vi "Error Handler Loop.vi"(8 "error in (no error)":errorcluster) -> (0 "error out":errorcluster)   [LabVIEW 2018, in "Error Handler.lvlib"]
uses:
  Error Handler.lvlib
  Q Ref FGV Command Enum.ctl
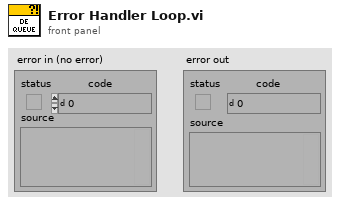
[diagram p1: front panel]
types:
  T1 = typedef "Error Handler.lvlib/Q Ref FGV Command Enum.ctl" = enum16{"Create Q", "Get Q", "Flush Q", "Release Q"}
  T2 = cluster{"Source":string, "Error to Handle":errorcluster}
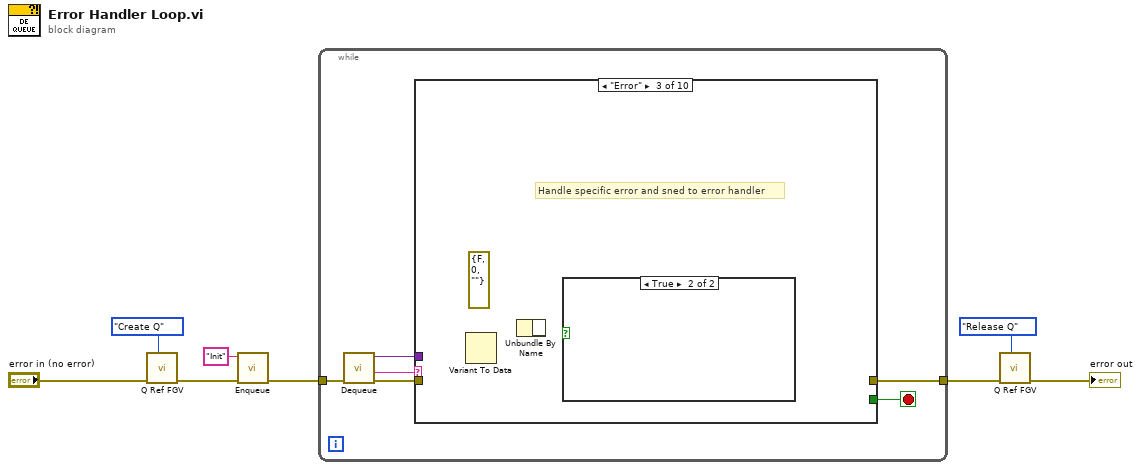
[diagram p0: block diagram]
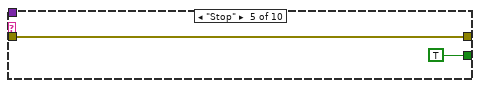
[diagram p6: hidden frame]
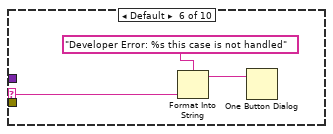
[diagram p7: hidden frame]
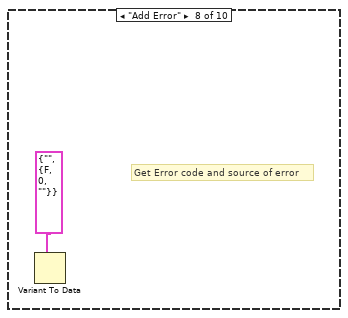
[diagram p9: hidden frame]
diagram:
  n1 = call "Q Ref FGV.vi"("Command"=Q_Ref_FGV_Command_Enum."Create Q", "error in (no error)"="error in (no error)") -> ("error out"=w5:errorcluster)  [unwired: 8 in, 1 out]
  n2 = call "Enqueue.vi"("error in (no error)"=w5, "Message"="Init") -> ("error out"=w3:errorcluster)  [unwired: 9 in]
  n3 = while {
    tunnel: w3 -> [w14]
    tunnel: [w9] -> w2
    stop <- w10 stop-if-true
    n4 = call "Dequeue.vi"("error in (no error)"=w14) -> ("error out"=w13:errorcluster, "Message"=w12:string, "Data"=w11:variant)  [unwired: 8 in]
    n5 = case shown="\"Error\"" w12 {
      selector: w12 -> [_ _ _ _ _ w18 _ _ _ _]
      tunnel: w13 -> [_ _ _ _ w15 _ _ _ _ _]
      tunnel: w11 -> [_ _ _ _ _ _ _ _ _ _]
      tunnel: [_ _ _ _ TRUE _ _ _ _ _] -> w10
      tunnel: [_ _ _ _ w15 _ _ _ _ _] -> w9
      frame "---- Framework Cases----" {
      }
      frame "Init" {
      }
      frame "Error" {
        (unwired) errorcluster {"status"=FALSE, "code"=0, "source"=""} ("error in (no error)")
        # "Handle specific error and sned to error handler"
        n6 = Variant To Data() -> ()  [unwired: 3 in, 2 out]
        n7 = Unbundle By Name() -> ()  [unwired: 1 in, 1 out]
        n8 = case shown="True" {
          selector: _ -> [_ _]
          frame False {
          }
          frame True {
          }
        }
      }
      frame "Timeout" {
      }
      frame "Stop" {
      }
      frame Default {
        n9 = Format Into String(format string="Developer Error: %s this case is not handled", w18) -> (resulting string=w19:string)  [unwired: 2 in, 1 out]
        n10 = One Button Dialog(message=w19) -> ()  [unwired: 1 in, 1 out]
      }
      frame "---- Public Message Cases ----" {
      }
      frame "Add Error" {
        # "Get Error code and source of error"
        n11 = Variant To Data(type=T2 {"Source"="", "Error to Handle"={"status"=FALSE, "code"=0, "source"=""}} ("output cluster")) -> ()  [unwired: 2 in, 2 out]
      }
      frame "---- Private Message Cases ----" {
      }
      frame "Log Error" {
        # "Log Error to disc"
      }
    }
  }
  n12 = call "Q Ref FGV.vi"("Command"=Q_Ref_FGV_Command_Enum."Release Q", "error in (no error)"=w2) -> ("error out"=→"error out":errorcluster)  [unwired: 8 in, 1 out]
